vi "get_number_of_scan_pixels.vi"(8 "error in (no error)":errorcluster, 11 "DL090201FrameScanTrajectory in":refnum<class "TrajectoryDL090201FrameScan.lvclass">) -> (0 "error out":errorcluster, 2 "number of scan pixels":i32, 3 "DL090201FrameScanTrajectory out":refnum<class "TrajectoryDL090201FrameScan.lvclass">)   [LabVIEW 2010, in "TrajectoryDL090201FrameScan.lvclass"]
uses:
  TrajectoryDL090201FrameScan.lvclass
  TrajectoryDL090201FrameScan.lvclass/TrajectoryDL090201FrameScan.ctl
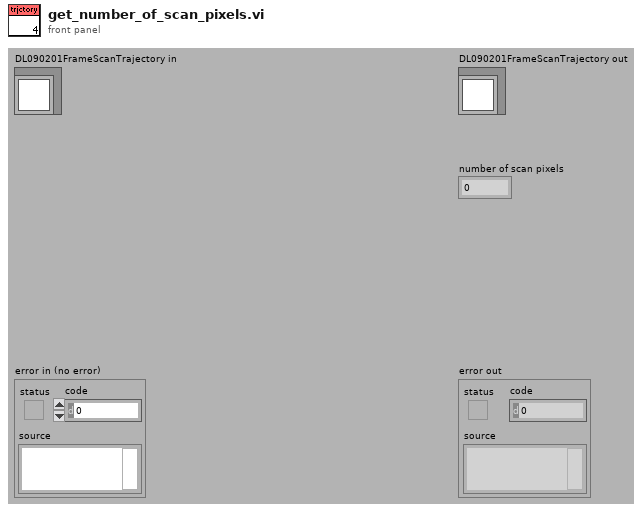
[diagram p1: front panel]
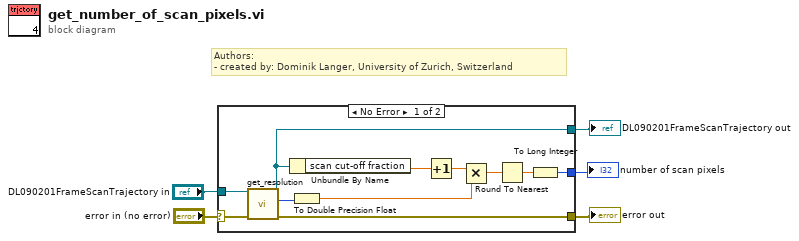
[diagram p0: block diagram]
diagram:
  # "Authors: \n- created by: Dominik Langer, University of Zurich, Switzerland"
  n1 = case shown="No Error" "error in (no error)" {
    selector: "error in (no error)" -> [w10 w18]
    tunnel: [w6 w18] -> w4
    tunnel: [w8 w17] -> w2
    tunnel: "DL090201FrameScanTrajectory in" -> [w9 w17]
    tunnel: [w14 _] -> w1
    frame No Error {
      n2 = call-dynamic "get_resolution.vi"("error in (no error)"=w10, "TrajectoryDL090201FrameScan in"=w9) -> ("error out"=w6:errorcluster, "x"=w7:i32, "TrajectoryDL090201FrameScan out"=w8:refnum<class "TrajectoryDL090201FrameScan.lvclass">)  [unwired: 7 out]
      n3 = Unbundle By Name(w8) -> ("scan cut-off fraction"=w12:dbl)
      n4 = To Double Precision Float(number=w7) -> (double precision float=w13:dbl)
      n5 = Increment(x=w12) -> (x+1=w11:dbl)
      n6 = Multiply(x=w11, y=w13) -> (x*y=w16:dbl)
      n7 = Round To Nearest(number=w16) -> (nearest integer value=w15:dbl)
      n8 = To Long Integer(number=w15) -> (32bit integer=w14:i32)
    }
    frame Error {
    }
  }
  "error out" <- w4
  "DL090201FrameScanTrajectory out" <- w2
  "number of scan pixels" <- w1
